vi "Configure Serial Output Channel.vi"(0 "channel source file paths":T2, 5 "fpga buffer start thresholds":T1={"timestamp buffer start threshold"=512, "packet data buffer start threshold (bytes)"=32768, "dram partition start threshold (bytes)"=2147483648}, 7 "dram partition size (bytes)":u64, 9 "packet timing error threshold (cycles)":u64=10, 11 "error in (no error)":errorcluster, 12 "enable i2c tap (all channels)":bool=TRUE, 13 "start trigger delay (cycles)":i64) -> (4 "datapath config":T3, 15 "error out":errorcluster)   [LabVIEW 2023, in "GettingStarted_Gen_148X_Host.lvlib"]
uses:
  GettingStarted_Gen_148X_Host.lvlib
  FPGA/Gen/Types/Serial Output Channel Datapath Configuration.ctl
  Types/Channel Source File Paths.ctl
  Types/FPGA Buffer Start Thresholds.ctl
  FPGA/Gen/GettingStarted_Gen_148X_FPGA.lvlib
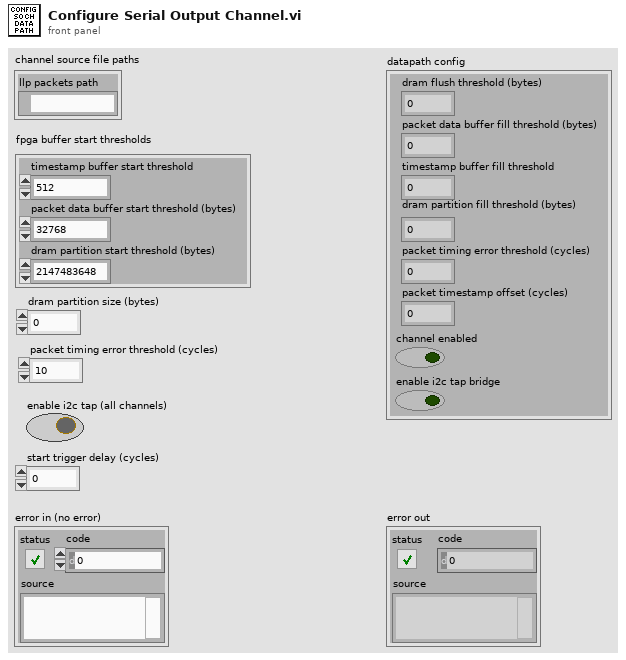
[diagram p1: front panel]
types:
  T1 = typedef "GettingStarted_Gen_148X_Host.lvlib/FPGA Buffer Start Thresholds.ctl" = cluster{"timestamp buffer start threshold":u32, "packet data buffer start threshold (bytes)":u64, "dram partition start threshold (bytes)":u64}
  T2 = typedef "GettingStarted_Gen_148X_Host.lvlib/Channel Source File Paths.ctl" = cluster{"llp packets path":path}
  T3 = typedef "GettingStarted_Gen_148X_FPGA.lvlib/Serial Output Channel Datapath Configuration.ctl" = cluster{"dram flush threshold (bytes)":u64, "packet data buffer fill threshold (bytes)":u64, "timestamp buffer fill threshold":u32, "packet timing error threshold (cycles)":u64, "channel enabled":bool, "dram partition fill threshold (bytes)":u64, "enable i2c tap bridge":bool, "packet timestamp offset (cycles)":i64}
  T4 = enum16{"open", "open or create", "create or replace", "create", "open (read-only)"}
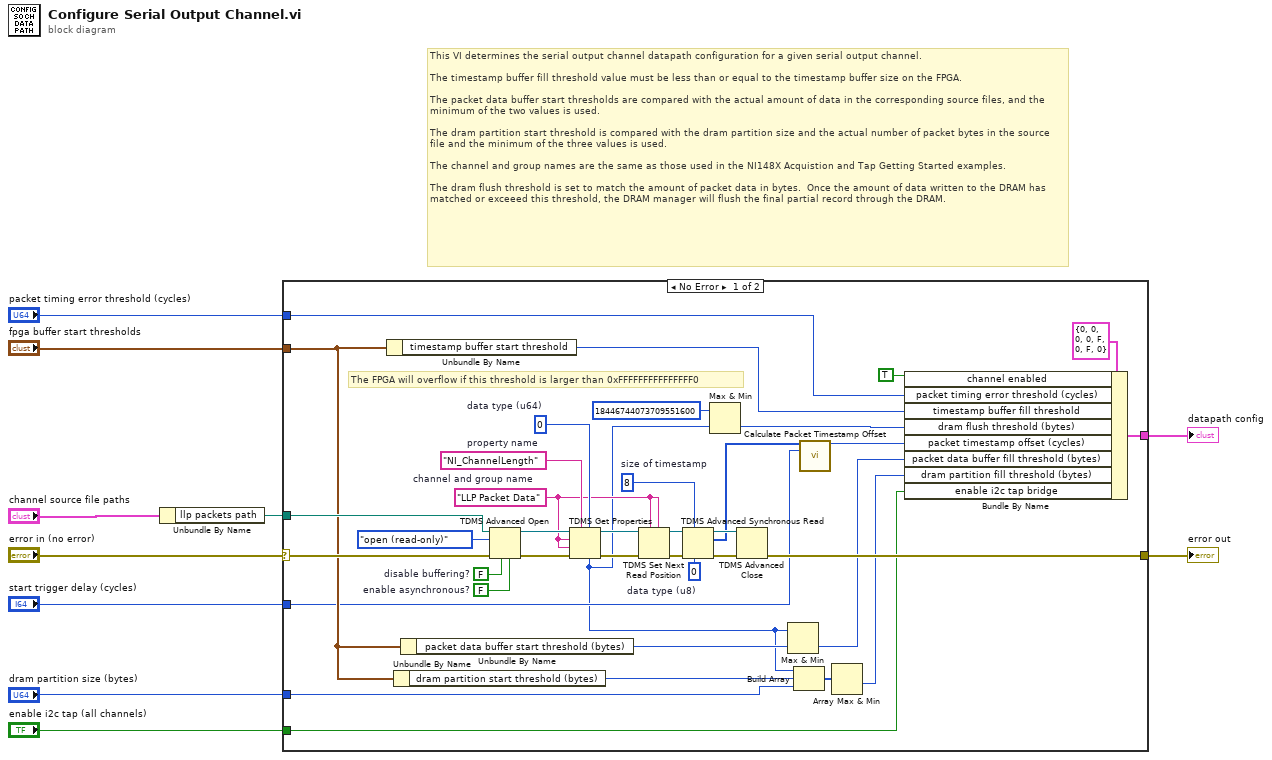
[diagram p0: block diagram]
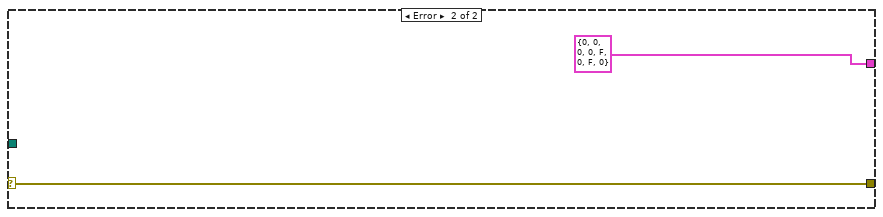
[diagram p2: hidden frame]
diagram:
  # "This VI determines the serial output channel datapath configuration for a given serial output channel.  \n\nThe timestamp buffer fill threshold value must be less than or equal to the timestamp buffer size on the FPGA.\n\nThe packet data buffer start thresholds are compared with the actual amount of data in the corresponding source files, and the minimum of the two values is used.  \n\nThe dram partition start threshold is compared with the dram partition size and the actual number of packet bytes in the source file and the minimum of the three values is used.\n\nThe channel and group names are the same as those used in the NI148X Acquistion and Tap Getting Started examples.\n\nThe dram flush threshold is set to match the amount of packet data in bytes.  Once the amount of data written to the DRAM has matched or exceeed this threshold, the DRAM manager will flush the final partial record through the DRAM."
  n1 = Unbundle By Name("channel source file paths") -> ("llp packets path"=w5:path)
  n2 = case shown="No Error" "error in (no error)" {
    selector: "error in (no error)" -> [w37 w50]
    tunnel: "packet timing error threshold (cycles)" -> [w40 _]
    tunnel: [w39 T3 {"dram flush threshold (bytes)"=0, "packet data buffer fill threshold (bytes)"=0, "timestamp buffer fill threshold"=0, "packet timing error threshold (cycles)"=0, "channel enabled"=FALSE, "dram partition fill threshold (bytes)"=0, "enable i2c tap bridge"=FALSE, "packet timestamp offset (cycles)"=0} ("datapath configs")] -> w9
    tunnel: [w38 w50] -> w8
    tunnel: w5 -> [w36 _]
    tunnel: "fpga buffer start thresholds" -> [w35 _]
    tunnel: "dram partition size (bytes)" -> [w34 _]
    tunnel: "enable i2c tap (all channels)" -> [w27 _]
    tunnel: "start trigger delay (cycles)" -> [w18 _]
    frame No Error {
      w14 = FALSE  # enable asynchronous?
      w17 = u8 0  # data type (u8)
      w23 = i64 8  # size of timestamp
      w43 = FALSE  # disable buffering?
      w45 = u64 0  # data type (u64)
      w47 = "NI_ChannelLength"  # property name
      w24 = "LLP Packet Data"  # channel and group name
      # "The FPGA will overflow if this threshold is larger than 0xFFFFFFFFFFFFFFF0"
      n3 = Unbundle By Name(w35) -> ("timestamp buffer start threshold"=w30:u32)
      n4 = Unbundle By Name(w35) -> ("dram partition start threshold (bytes)"=w33:u64)
      n5 = Unbundle By Name(w35) -> ("packet data buffer start threshold (bytes)"=w29:u64)
      n6 = TDMS Advanced Open(4:w14, 6:w43, 8:w37, 10:T4."open (read-only)" ("operation (0:open)"), 11:w36) -> (0:w44:errorcluster, 3:w46:refnum<k34>)  [unwired: 1 out]
      n7 = TDMS Get Properties(5:w45, 7:w47, 8:w44, 9:w24, 10:w24, 11:w46) -> (0:w26:errorcluster, 3:w25:refnum<k34>, 4:w12:u64)  [unwired: 3 out]
      n8 = TDMS Set Next Read Position(5:w24, 7:w24, 8:w26, 11:w25) -> (0:w16:errorcluster, 3:w15:refnum<k34>)  [unwired: 2 in]
      n9 = TDMS Advanced Synchronous Read(6:w17, 7:w23, 8:w16, 11:w15) -> (0:w21:errorcluster, 2:w20:u8[], 3:w22:refnum<k34>)  [unwired: 1 out]
      n10 = Max & Min(x=u64 18446744073709551600, y=w12) -> (min(x,y)=w11:u64)  [unwired: 1 out]
      n11 = TDMS Advanced Close(8:w21, 11:w22) -> (0:w38:errorcluster)  [unwired: 2 in, 1 out]
      n12 = Max & Min(x=w12, y=w29) -> (min(x,y)=w28:u64)  [unwired: 1 out]
      n13 = Build Array(w12, w33, w34) -> (w32:u64[])
      n14 = call "Calculate Packet Timestamp Offset.vi"("first packet timestamp (bytes)"=w20, "start trigger delay (s)"=w18) -> ("packet timestamp offset"=w19:i64)  [unwired: 13 in]
      n15 = Array Max & Min(array=w32) -> (min value=w31:u64)  [unwired: 3 out]
      n16 = Bundle By Name(cluster=T3 {"dram flush threshold (bytes)"=0, "packet data buffer fill threshold (bytes)"=0, "timestamp buffer fill threshold"=0, "packet timing error threshold (cycles)"=0, "channel enabled"=FALSE, "dram partition fill threshold (bytes)"=0, "enable i2c tap bridge"=FALSE, "packet timestamp offset (cycles)"=0} ("datapath configs"), "channel enabled"=TRUE, "packet timing error threshold (cycles)"=w40, "timestamp buffer fill threshold"=w30, "dram flush threshold (bytes)"=w11, "packet timestamp offset (cycles)"=w19, "packet data buffer fill threshold (bytes)"=w28, "dram partition fill threshold (bytes)"=w31, "enable i2c tap bridge"=w27) -> (w39:T3)
    }
    frame Error {
    }
  }
  "datapath config" <- w9
  "error out" <- w8
